vi "DAQDeviceReset.vi"() -> ()   [LabVIEW 2011]
panel:
  in  "device in":tag
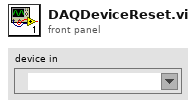
[diagram p1: front panel]
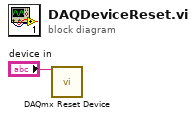
[diagram p0: block diagram]
diagram:
  n1 = call <vilib>:"DAQmx Reset Device.vi"("device in"="device in") -> ()  [unwired: 14 in, 1 out]
